vi "Bundle RT Configuration.vi"(8 "error in (no error)":errorcluster) -> (0 "error out":errorcluster, 3 "All Control Configuration Values":T1={"Control State"=enum."Safe State", "Setpoints"={"Channel 0"=0.0, "Channel 1"=0.0, "Channel 2"=0.0, "Channel 3"=0.0}, "Control Configurations"=[{"PID Gains"={"proportional gain (Kc)"=1.0, "integral gain (Kc*Ts/Ti)"=0.1, "derivative gain (Kc*Td/Ts)"=0.0}, "Output Range"={"output high"=5.0, "output low"=-5.0}}, {"PID Gains"={"proportional gain (Kc)"=1.0, "integral gain (Kc*Ts/Ti)"=0.1, "derivative gain (Kc*Td/Ts)"=0.0}, "Output Range"={"output high"=5.0, "output low"=-5.0}}, {"PID Gains"={"proportional gain (Kc)"=1.0, "integral gain (Kc*Ts/Ti)"=0.1, "derivative gain (Kc*Td/Ts)"=0.0}, "Output Range"={"output high"=5.0, "output low"=-5.0}}, {"PID Gains"={"proportional gain (Kc)"=1.0, "integral gain (Kc*Ts/Ti)"=0.1, "derivative gain (Kc*Td/Ts)"=0.0}, "Output Range"={"output high"=5.0, "output low"=-5.0}}], "Temperature Thresholds"=[20.0]} {"Control Configurations"."Output Range"."output high" min=-5.0 max=5.0})   [LabVIEW 2017]
uses:
  controls/All Control Configuration Values.ctl
  controls/Control State.ctl
  controls/Raw Values.ctl
  controls/Control Configuration.ctl
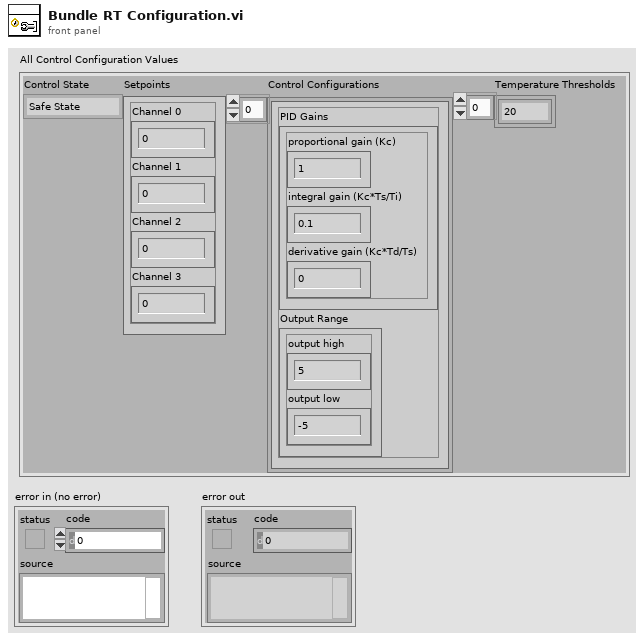
[diagram p1: front panel]
types:
  T1 = typedef "All Control Configuration Values.ctl" = cluster{"Control State":T2, "Setpoints":T3, "Control Configurations":T4[], "Temperature Thresholds":dbl[]}
  T2 = typedef "Control State.ctl" = enum16{"Safe State", "Control (PID)"}
  T3 = typedef "Raw Values.ctl" = cluster{"Channel 0":dbl, "Channel 1":dbl, "Channel 2":dbl, "Channel 3":dbl}
  T4 = typedef "Control Configuration.ctl" = cluster{"PID Gains":cluster{"proportional gain (Kc)":dbl, "integral gain (Kc*Ts/Ti)":dbl, "derivative gain (Kc*Td/Ts)":dbl}, "Output Range":cluster{"output high":dbl, "output low":dbl}}
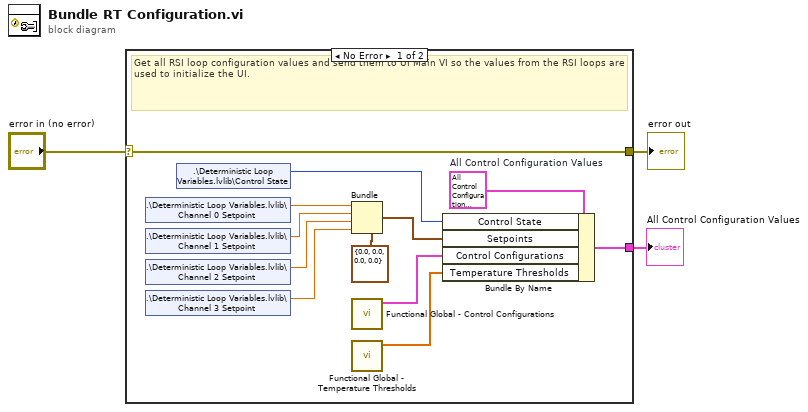
[diagram p0: block diagram]
diagram:
  n1 = case shown="No Error" "error in (no error)" {
    selector: "error in (no error)" -> [w14 w16]
    tunnel: [w14 w16] -> w2
    tunnel: [w15 _] -> w1
    frame No Error {
      w5 = T1 {"Control State"=enum."Safe State", "Setpoints"={"Channel 0"=0.0, "Channel 1"=0.0, "Channel 2"=0.0, "Channel 3"=0.0}, "Control Configurations"=[], "Temperature Thresholds"=[]}  # All Control Configuration Values
      # "Get all RSI loop configuration values and send them to UI Main VI so the values from the RSI loops are used to initialize the UI."
      n2 = shared-variable ".\\Deterministic Loop Variables.lvlib\\Channel 0 Setpoint"() -> (w9:dbl)  [unwired: 1 in, 1 out]
      n3 = shared-variable ".\\Deterministic Loop Variables.lvlib\\Channel 1 Setpoint"() -> (w8:dbl)  [unwired: 1 in, 1 out]
      n4 = shared-variable ".\\Deterministic Loop Variables.lvlib\\Channel 2 Setpoint"() -> (w7:dbl)  [unwired: 1 in, 1 out]
      n5 = shared-variable ".\\Deterministic Loop Variables.lvlib\\Channel 3 Setpoint"() -> (w6:dbl)  [unwired: 1 in, 1 out]
      n6 = shared-variable ".\\Deterministic Loop Variables.lvlib\\Control State"() -> (w10:T2)  [unwired: 1 in, 1 out]
      n7 = Bundle(cluster=T3 {"Channel 0"=0.0, "Channel 1"=0.0, "Channel 2"=0.0, "Channel 3"=0.0} ("Raw Values"), "Channel 0"=w9, "Channel 1"=w8, "Channel 2"=w7, "Channel 3"=w6) -> (w13:T3)
      n8 = call "Functional Global - Control Configurations.vi"() -> ("Control Configurations out"=w4:T4[])  [unwired: 11 in]
      n9 = call "Functional Global - Temperature Thresholds.vi"() -> ("Temperature Thresholds out"=w11:dbl[])  [unwired: 11 in]
      n10 = Bundle By Name(cluster=w5, "Control State"=w10, "Setpoints"=w13, "Control Configurations"=w4, "Temperature Thresholds"=w11) -> (w15:T1)
    }
    frame Error {
      # "Error"
    }
  }
  "error out" <- w2
  "All Control Configuration Values" <- w1
